vi "avg256.vi"(10 "Input":i16) -> (2 "Output":i16)   [LabVIEW 2011, in "kevLib2011.lvlib"]
uses:
  kevLib2011.lvlib
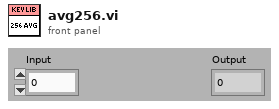
[diagram p1: front panel]
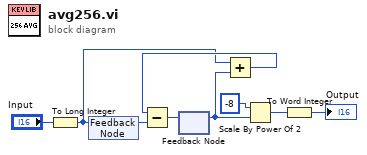
[diagram p0: block diagram]
diagram:
  n1 = To Long Integer(number="Input") -> (32bit integer=w4:i32)
  n2 = feedback-in #1(w4) -> ()
  n3 = feedback #1() -> (w1:i32)  [unwired: 1 in]
  n4 = feedback #2() -> (w7:i32)  [unwired: 1 in]
  n5 = Add(x=w4, y=w7) -> (x+y=w9:i32)
  n6 = Subtract(x=w9, y=w1) -> (x-y=w8:i32)
  n7 = feedback-in #2(w8) -> ()
  n8 = Scale By Power Of 2(n=-8, x=w7) -> (x*2^n=w3:i32)
  n9 = To Word Integer(number=w3) -> (16bit integer=→"Output":i16)
